vi "LViradon.vi"() -> ()   [LabVIEW 2018]
uses:
  <vilib>/Utility/file.llb/Read Delimited Spreadsheet (DBL).vi
panel:
  out "path":path
  in  "Read Directory":string
  out "Recon":T1(plugin-control)
  out "Sinogram":T1(plugin-control)
  in  "N_det":dbl=40.0
  in  "N_rot":dbl=40.0
  out "error out 2":errorcluster
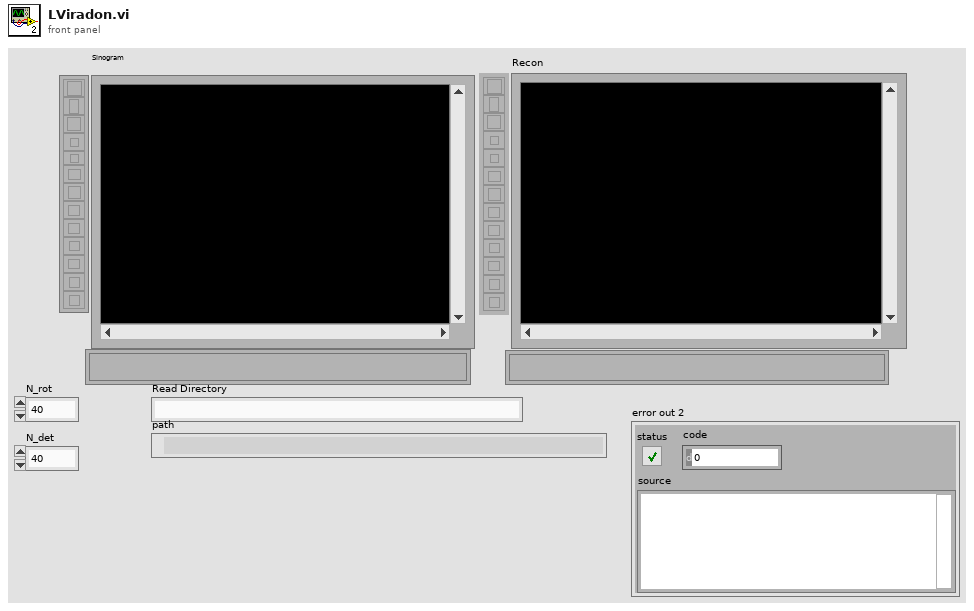
[diagram p1: front panel]
types:
  T1 = typedef "IMAQ Image.ctl" = refnum<image>
  T2 = typedef "Image Type" = u32
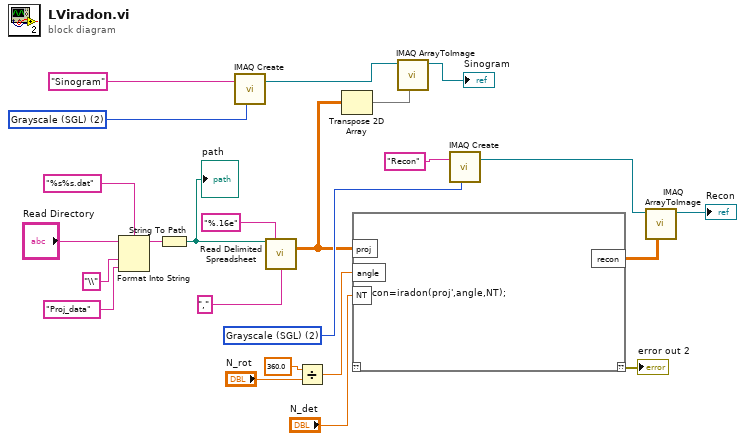
[diagram p0: block diagram]
diagram:
  w14 = T2 2 items=["Grayscale (U8)", "Grayscale (I16)", "Grayscale (SGL)", "Complex (CSG)", "RGB (U32)", "HSL (U32)", "RGB (U64)", "Grayscale (U16)"] ("Image Type")
  w12 = T2 2 items=["Grayscale (U8)", "Grayscale (I16)", "Grayscale (SGL)", "Complex (CSG)", "RGB (U32)", "HSL (U32)", "RGB (U64)", "Grayscale (U16)"] ("Image Type")
  n1 = Format Into String(format string="%s%s.dat", initial string="Read Directory", "\\" ("input 1"), "Proj_data" ("input 2")) -> (resulting string=w23:string)  [unwired: 1 in, 1 out]
  n2 = String To Path(string=w23) -> (path=w19:path)
  "path" <- w19
  n3 = call "IMAQ Create"("Image Name"="Sinogram", "Image Type"=w12) -> ("New Image"=w13:T1)  [unwired: 3 in, 1 out]
  n4 = call-poly <vilib>:"Read Delimited Spreadsheet.vi"("file path (dialog if empty)"=w19, "format (%.3f)"="%.16e", "delimiter (\\t)"="," ("delimiter (\\t)")) -> ("all rows"=w6:dbl[][])  [unwired: 7 in, 5 out]
  n5 = Divide(x=360.0, y="N_rot") -> (x/y=w9:dbl)
  n6 = Transpose 2D Array(2D array=w6) -> (transposed array=w7:dbl[][])
  n7 = script code="recon=iradon(proj',angle,NT);"("proj"=w6, "angle"=w9, "NT"="N_det") -> ("??"=→"error out 2":errorcluster, "recon"=w16:dbl[][])  [unwired: 1 in]
  n8 = call "IMAQ ArrayToImage"("Image Pixels (Float)"=w7, "Image"=w13) -> ("Image Out"=→"Sinogram":T1)  [unwired: 8 in, 1 out]
  n9 = call "IMAQ Create"("Image Name"="Recon", "Image Type"=w14) -> ("New Image"=w15:T1)  [unwired: 3 in, 1 out]
  n10 = call "IMAQ ArrayToImage"("Image Pixels (Float)"=w16, "Image"=w15) -> ("Image Out"=→"Recon":T1)  [unwired: 8 in, 1 out]
